vi "LVClass_HasoSlopes to XML string format.vi"(0 "HasoSlopes in":refnum<class "HasoSlopes.lvclass">, 11 "error in (no error)":errorcluster) -> (4 "HasoSlopes out":refnum<class "HasoSlopes.lvclass">, 6 "XML string format":string, 15 "error out":errorcluster)   [LabVIEW 2020, in "HasoSlopes.lvclass"]
doc: "int32_t Imop_HasoSlopes_SlopesY(CStr message, int32_t objet, float *Slopesy);"
uses:
  HasoSlopes.lvclass
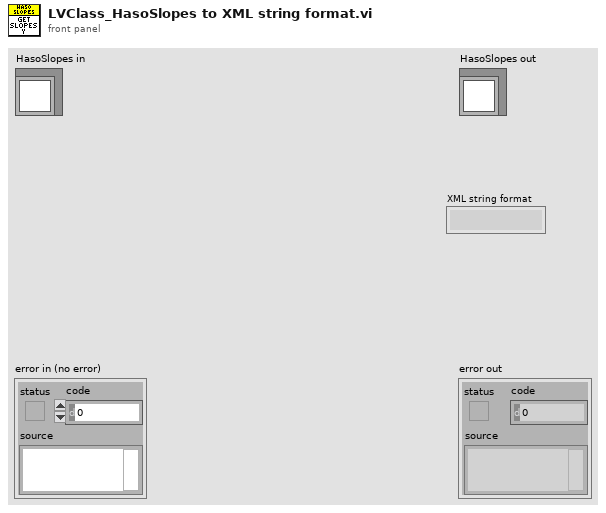
[diagram p1: front panel]
types:
  T1 = cluster{"second":i32, "minute":i32, "hour":i32, "day of month":i32, "month":i32, "year":i32, "day of week":i32, "day of year":i32, "is DST":i32}
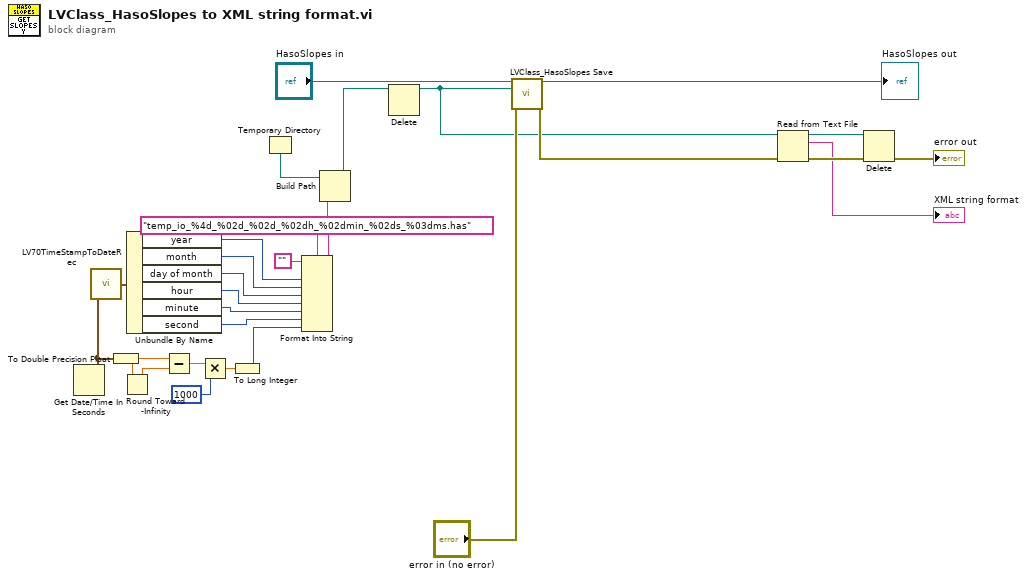
[diagram p0: block diagram]
diagram:
  n1 = Get Date/Time In Seconds() -> (seconds since 1Jan1904=w22:timestamp)
  n2 = call <vilib>:"LV70TimeStampToDateRec.vi"("time stamp"=w22) -> ("date time rec"=w23:T1)
  n3 = To Double Precision Float(number=w22) -> (double precision float=w21:dbl)
  n4 = Round Toward -Infinity(1:w21) -> (0:w20:dbl)
  n5 = Unbundle By Name(w23) -> ("year"=w13:i32, "month"=w14:i32, "day of month"=w12:i32, "hour"=w11:i32, "minute"=w10:i32, "second"=w9:i32)
  n6 = Subtract(x=w21, y=w20) -> (x-y=w19:dbl)
  n7 = Multiply(x=w19, y=1000) -> (x*y=w17:dbl)
  n8 = To Long Integer(number=w17) -> (32bit integer=w8:i32)
  n9 = Temporary Directory() -> (w24:path)
  n10 = Format Into String(format string="temp_io_%4d_%02d_%02d_%02dh_%02dmin_%02ds_%03dms.has", initial string="", w13, w14, w12, w11, w10, w9, w8) -> (resulting string=w7:string)  [unwired: 1 in, 1 out]
  n11 = Build Path(base path=w24, name or relative path=w7) -> (appended path=w6:path)
  n12 = Delete(path (use dialog)=w6) -> (deleted path=w4:path)  [unwired: 4 in, 2 out]
  n13 = call "LVClass_HasoSlopes Save.vi"("HasoSlopes in"="HasoSlopes in", "path"=w4, "error in (no error)"="error in (no error)") -> ("HasoSlopes out"=→"HasoSlopes out":refnum<class "HasoSlopes.lvclass">, "error out"=w5:errorcluster)  [unwired: 11 in]
  n14 = Read from Text File(file (use dialog)=w4, error in=w5) -> (text=→"XML string format":string, error out=w3:errorcluster)  [unwired: 2 in, 2 out]
  n15 = Delete(path (use dialog)=w4, error in=w3) -> (error out=→"error out":errorcluster)  [unwired: 3 in, 2 out]
